vi "Begin.vi"(8 "error in":errorcluster) -> (0 "error out":errorcluster)   [LabVIEW 2014]
doc: "Called before other user functions, this VI is expected to open initial I/O refnums, load in file data, and do all program initialization. Notice that the <B>error out</B> terminal is simply used for data flow. Wiring it to other structures or subVIs ensures that this VI runs first."
uses:
  <vilib>/Rock Robotics/WPI/SafetyOutput/WPI_SafetyOutputConfigMenu.ctl
  <vilib>/Rock Robotics/SystemInterfaces/DIO/FPGA_DIOPWMChannel.ctl
  <vilib>/Rock Robotics/WPI/Joystick/WPI_JoystickDeviceEnum.ctl
  <vilib>/Rock Robotics/WPI/RobotDrive/WPI_RobotDriveOpen4MotorWithCANTalonSRX.vi
  <vilib>/Rock Robotics/WPI/MotorControl/WPI_MotorControlOpen Talon.vi
  <vilib>/Rock Robotics/WPI/MotorControl/WPI_MotorControlOpenCANTalonSRX.vi
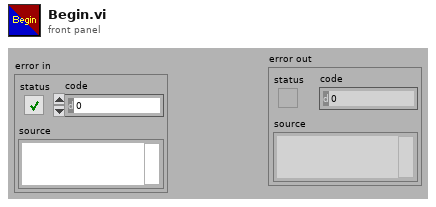
[diagram p1: front panel]
types:
  T1 = typedef "WPI_SafetyOutputConfigMenu.ctl" = enum16{"Enable", "Disable"}
  T2 = typedef "WPI_RobotDriveDevRef.ctl" = cluster{"DevStatus":errorcluster, "Motors[]":T3[], "Square Inputs":bool, "Max Output":dbl}
  T3 = typedef "WPI_MotorControlDeviceRef.ctl" = cluster{"DeviceStatus":errorcluster, "Type":T4, "PWM":cluster{"Controller":T5, "PWM Channel":T6, "DeadBand":T7}, "CAN":cluster{"Device Number":u8, "Control Mode":T8, "Semaphore":T9, "Max Vout":dbl, "TalonSRX Control Mode":T10}, "Invert":bool, "TransformRef":T11, "InvTransformRef":T11}
  T4 = typedef "WPI_MotorControlType.ctl" = enum16{"PWM", "CAN", "CANTalonSRX"}
  T5 = typedef "FPGA_TypedefDigitalModule.ctl" = enum16{"Controller 1"}
  T6 = typedef "FPGA_DIOPWMChannel.ctl" = enum8{"PWM 0", "PWM 1", "PWM 2", "PWM 3", "PWM 4", "PWM 5", "PWM 6", "PWM 7", "PWM 8", "PWM 9", "PWM MXP 0", "PWM MXP 1", "PWM MXP 2", "PWM MXP 3", "PWM MXP 4", "PWM MXP 5", "PWM MXP 6", "PWM MXP 7", "PWM MXP 8", "PWM MXP 9", "Invalid"}
  T7 = typedef "WPI_PWMDeadband.ctl" = cluster{"Name":string, "maxPositivePwm":i32, "minPositivePwm":i32, "centerPwm":i32, "maxNegativePwm":i32, "minNegativePwm":i32, "angularRange":u16}
  T8 = typedef "WPI_CANJaguar_ControlMode.ctl" = enum8{"Percent VBus", "Current", "Speed", "Position", "Voltage"}
  T9 = typedef "Semaphore RefNum" = refnum<k1>
  T10 = typedef "WPI_CANTalonSRX_APIControlMode.ctl" = enum8{"Percent VBus", "Speed", "Position", "Slave", "Unchanged / Invalid"}
  T11 = typedef "WPI_PWMTransform_ConPane.ctl" = refnum<vi>
  T12 = typedef "WPI_JoystickDeviceEnum.ctl" = enum16{"USB 0", "USB 1", "USB 2", "USB 3", "USB 4", "USB 5"}
  T13 = typedef "WPI_JoystickDevRef.ctl" = cluster{"Device":T12}
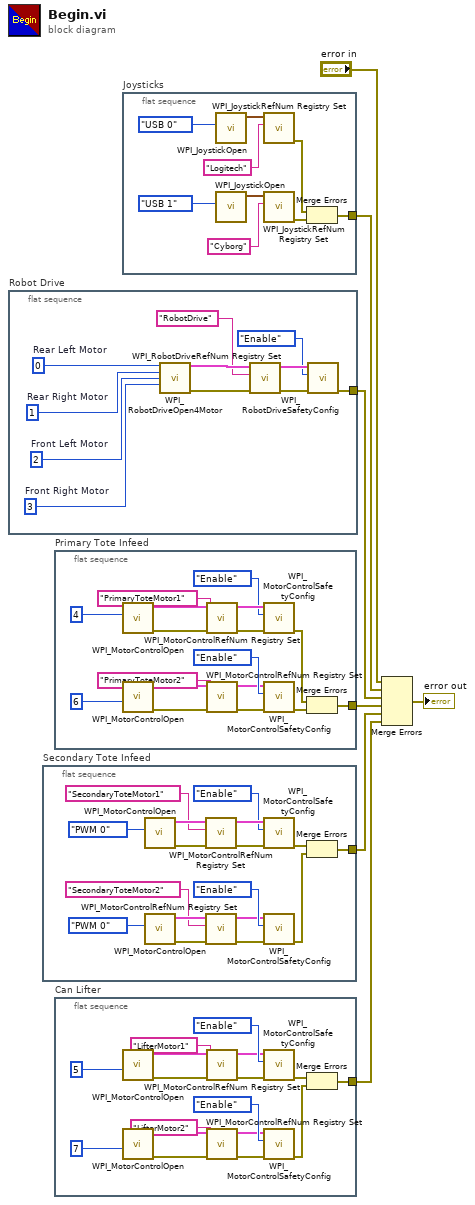
[diagram p0: block diagram]
diagram:
  n1 = flat-sequence "Robot Drive" {
    tunnel: [w8] -> w7
    frame #0 {
      w15 = u8 3  # Front Right Motor
      w16 = u8 2  # Front Left Motor
      w17 = u8 1  # Rear Right Motor
      w18 = u8 0  # Rear Left Motor
      n2 = call-poly <vilib>:"WPI_RobotDriveOpen4Motor.vi"("Rear Left Motor"=w18, "Rear Right Motor"=w17, "Front Left Motor"=w16, "Front Right Motor"=w15) -> ("RobotDriveDevRef"=w14:T2, "error out"=w13:errorcluster)  [unwired: 10 in]
      n3 = call <vilib>:"WPI_RobotDriveRefNum Registry Set.vi"("error in (no error)"=w13, "refnum name"="RobotDrive", "RobotDriveDevRef"=w14) -> ("error out"=w10:errorcluster, "RobotDriveDevRef"=w11:T2)  [unwired: 7 in]
      n4 = call <vilib>:"WPI_RobotDriveSafetyConfig.vi"("error in (no error)"=w10, "mode"=WPI_SafetyOutputConfigMenu."Enable", "RobotDriveDevRef"=w11) -> ("error out"=w8:errorcluster)  [unwired: 7 in, 1 out]
    }
  }
  n5 = flat-sequence "Secondary Tote Infeed" {
    tunnel: [w19] -> w4
    frame #0 {
      n6 = call-poly <vilib>:"WPI_MotorControlOpen.vi"("PWM Channel"=FPGA_DIOPWMChannel."PWM 0") -> ("error out"=w30:errorcluster, "MotorControlDeviceRef"=w31:T3)  [unwired: 9 in]
      n7 = call-poly <vilib>:"WPI_MotorControlOpen.vi"("PWM Channel"=FPGA_DIOPWMChannel."PWM 0") -> ("error out"=w24:errorcluster, "MotorControlDeviceRef"=w25:T3)  [unwired: 9 in]
      n8 = call <vilib>:"WPI_MotorControlRefNum Registry Set.vi"("error in (no error)"=w30, "refnum name"="SecondaryToteMotor1", "MotorControlDevRef"=w31) -> ("error out"=w33:errorcluster, "MotorControlDevRef"=w32:T3)  [unwired: 7 in]
      n9 = call <vilib>:"WPI_MotorControlRefNum Registry Set.vi"("error in (no error)"=w24, "refnum name"="SecondaryToteMotor2", "MotorControlDevRef"=w25) -> ("error out"=w26:errorcluster, "MotorControlDevRef"=w27:T3)  [unwired: 7 in]
      n10 = call <vilib>:"WPI_MotorControlSafetyConfig.vi"("error in (no error)"=w33, "mode"=WPI_SafetyOutputConfigMenu."Enable", "MotorControlDevRef"=w32) -> ("error out"=w21:errorcluster)  [unwired: 7 in, 1 out]
      n11 = call <vilib>:"WPI_MotorControlSafetyConfig.vi"("error in (no error)"=w26, "mode"=WPI_SafetyOutputConfigMenu."Enable", "MotorControlDevRef"=w27) -> ("error out"=w20:errorcluster)  [unwired: 7 in, 1 out]
      n12 = Merge Errors(w21, w20) -> (w19:errorcluster)
    }
  }
  n13 = flat-sequence "Primary Tote Infeed" {
    tunnel: [w38] -> w5
    frame #0 {
      n14 = call-poly <vilib>:"WPI_MotorControlOpen.vi"("Device Number"=u8 4) -> ("error out"=w50:errorcluster, "MotorControlDeviceRef"=w49:T3)  [unwired: 9 in]
      n15 = call-poly <vilib>:"WPI_MotorControlOpen.vi"("Master Device Number"=u8 6) -> ("error out"=w48:errorcluster, "MotorControlDeviceRef"=w47:T3)  [unwired: 9 in]
      n16 = call <vilib>:"WPI_MotorControlRefNum Registry Set.vi"("error in (no error)"=w50, "refnum name"="PrimaryToteMotor1", "MotorControlDevRef"=w49) -> ("error out"=w45:errorcluster, "MotorControlDevRef"=w46:T3)  [unwired: 7 in]
      n17 = call <vilib>:"WPI_MotorControlRefNum Registry Set.vi"("error in (no error)"=w48, "refnum name"="PrimaryToteMotor2", "MotorControlDevRef"=w47) -> ("error out"=w42:errorcluster, "MotorControlDevRef"=w41:T3)  [unwired: 7 in]
      n18 = call <vilib>:"WPI_MotorControlSafetyConfig.vi"("error in (no error)"=w45, "mode"=WPI_SafetyOutputConfigMenu."Enable", "MotorControlDevRef"=w46) -> ("error out"=w40:errorcluster)  [unwired: 7 in, 1 out]
      n19 = call <vilib>:"WPI_MotorControlSafetyConfig.vi"("error in (no error)"=w42, "mode"=WPI_SafetyOutputConfigMenu."Enable", "MotorControlDevRef"=w41) -> ("error out"=w39:errorcluster)  [unwired: 7 in, 1 out]
      n20 = Merge Errors(w40, w39) -> (w38:errorcluster)
    }
  }
  n21 = flat-sequence "Can Lifter" {
    tunnel: [w55] -> w3
    frame #0 {
      n22 = call-poly <vilib>:"WPI_MotorControlOpen.vi"("Master Device Number"=u8 5) -> ("error out"=w67:errorcluster, "MotorControlDeviceRef"=w66:T3)  [unwired: 9 in]
      n23 = call-poly <vilib>:"WPI_MotorControlOpen.vi"("Master Device Number"=u8 7) -> ("error out"=w65:errorcluster, "MotorControlDeviceRef"=w64:T3)  [unwired: 9 in]
      n24 = call <vilib>:"WPI_MotorControlRefNum Registry Set.vi"("error in (no error)"=w67, "refnum name"="LifterMotor1", "MotorControlDevRef"=w66) -> ("error out"=w62:errorcluster, "MotorControlDevRef"=w61:T3)  [unwired: 7 in]
      n25 = call <vilib>:"WPI_MotorControlRefNum Registry Set.vi"("error in (no error)"=w65, "refnum name"="LifterMotor2", "MotorControlDevRef"=w64) -> ("error out"=w59:errorcluster, "MotorControlDevRef"=w58:T3)  [unwired: 7 in]
      n26 = call <vilib>:"WPI_MotorControlSafetyConfig.vi"("error in (no error)"=w62, "mode"=WPI_SafetyOutputConfigMenu."Enable", "MotorControlDevRef"=w61) -> ("error out"=w57:errorcluster)  [unwired: 7 in, 1 out]
      n27 = call <vilib>:"WPI_MotorControlSafetyConfig.vi"("error in (no error)"=w59, "mode"=WPI_SafetyOutputConfigMenu."Enable", "MotorControlDevRef"=w58) -> ("error out"=w56:errorcluster)  [unwired: 7 in, 1 out]
      n28 = Merge Errors(w57, w56) -> (w55:errorcluster)
    }
  }
  n29 = flat-sequence "Joysticks" {
    tunnel: [w70] -> w6
    frame #0 {
      n30 = call <vilib>:"WPI_JoystickOpen.vi"("JoystickDevice"=WPI_JoystickDeviceEnum."USB 0") -> ("JoystickDevRef"=w73:T13)  [unwired: 10 in]
      n31 = call <vilib>:"WPI_JoystickOpen.vi"("JoystickDevice"=WPI_JoystickDeviceEnum."USB 1") -> ("JoystickDevRef"=w76:T13)  [unwired: 10 in]
      n32 = call <vilib>:"WPI_JoystickRefNum Registry Set.vi"("refnum name"="Logitech", "JoystickDevRef"=w73) -> ("error out"=w72:errorcluster)  [unwired: 8 in, 1 out]
      n33 = call <vilib>:"WPI_JoystickRefNum Registry Set.vi"("refnum name"="Cyborg", "JoystickDevRef"=w76) -> ("error out"=w71:errorcluster)  [unwired: 8 in, 1 out]
      n34 = Merge Errors(w72, w71) -> (w70:errorcluster)
    }
  }
  n35 = Merge Errors("error in", w6, w7, w5, w4, w3) -> (→"error out":errorcluster)
